vi "error_message.vi"(8 "error in":errorcluster, 10 "Type of Dialog":T1(ring) caption="Type of Dialog (1: OK Msg)", 11 "VISA resource name":refnum<visa-resource-name>) -> (0 "error out":errorcluster, 1 "error message":string, 2 "error code (0)":i32 format="%.0x", 3 "VISA resource name out":refnum<visa-resource-name> caption="VISA resource name", 5 "Status":bool)   [LabVIEW 2014, in "rszvl_rsidr_core.lvlib"]
uses:
  rszvl_rsidr_core.lvlib
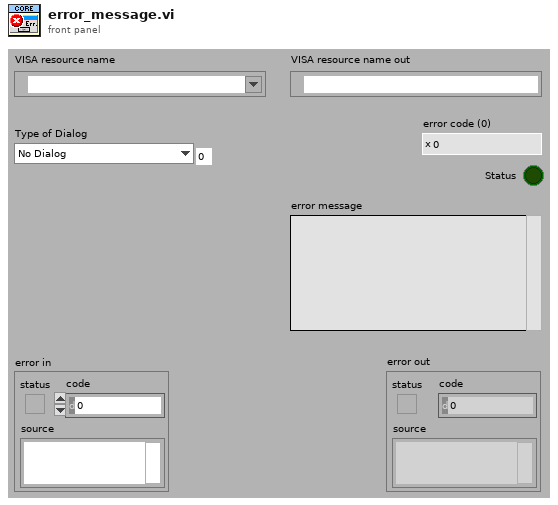
[diagram p1: front panel]
types:
  T1 = enum16{"No Dialog", "OK Message", "Continue or Stop Message"}
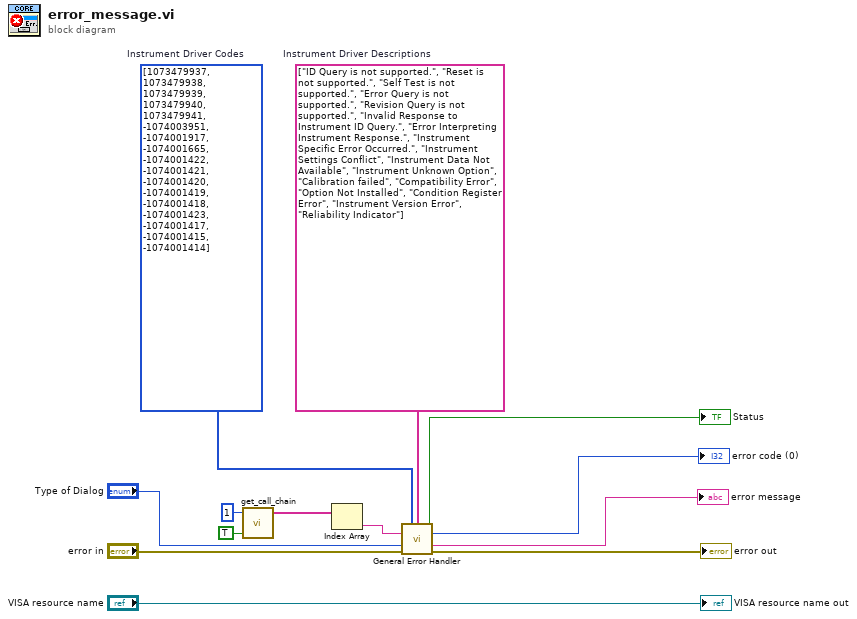
[diagram p0: block diagram]
diagram:
  w1 = i32[] [1073479937, 1073479938, 1073479939, 1073479940, 1073479941, -1074003951, -1074001917, -1074001665, -1074001422, -1074001421, -1074001420, -1074001419, -1074001418, -1074001423, -1074001417, -1074001415, -1074001414]  # Instrument Driver Codes
  w2 = string[] ["ID Query is not supported.", "Reset is not supported.", "Self Test is not supported.", "Error Query is not supported.", "Revision Query is not supported.", "Invalid Response to Instrument ID Query.", "Error Interpreting Instrument Response.", "Instrument Specific Error Occurred.", "Instrument Settings Conflict", "Instrument Data Not Available", "Instrument Unknown Option", "Calibration failed", "Compatibility Error", "Option Not Installed", "Condition Register Error", "Instrument Version Error", "Reliability Indicator"]  # Instrument Driver Descriptions
  n1 = call "get_call_chain.vi"("Remove lvlib names (F)"=TRUE, "Cut first x elements\nfrom Error Chain (0)"=1 ("Cut first x elements\nfrom Error Chain (0)")) -> ("Call chain out"=w4:string[])  [unwired: 1 in, 2 out]
  n2 = Index Array(array=w4) -> (element=w3:string)  [unwired: 1 in]
  n3 = call "General Error Handler.vi"("[user-defined codes]"=w1, "[user-defined descriptions]"=w2, "[error source] (\" \")"=w3, "type of dialog (OK msg:1)"="Type of Dialog", "error in (no error)"="error in") -> ("error?"=→"Status":bool, "code out"=→"error code (0)":i32, "message"=→"error message":string, "error out"=→"error out":errorcluster)  [unwired: 6 in, 1 out]
  "VISA resource name out" <- "VISA resource name"
